vi "LtaSet.vi"(8 "Error In":errorcluster[](array[cluster]), 10 "Data":variant) -> (0 "Error Out":errorcluster[](array[cluster]), 2 "BusNum":i32)   [LabVIEW 2014, in "Bus_class.lvlib" / "Bus.lvclass"]
uses:
  Bus.lvclass
  TestAutomation/Comms/CommsData.ctl
  <vilib>/Utility/error.llb/Error Cluster From Error Code.vi
  <vilib>/ErrorRing/Error Ring.xnode
  TestAutomation/Comms/Comms.lvlib
  <userlib>/NIST/NISTErrorLib/NISTErrorLib.lvlib
  TestAutomation/LTA/LTA.lvlib
  Framework.lvlib
panel:
  out "XMLData":string
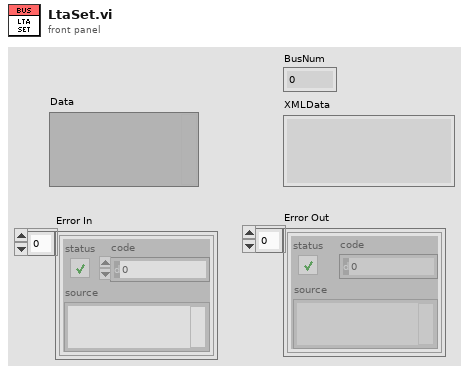
[diagram p1: front panel]
types:
  T1 = typedef "Comms.lvlib/CommsData.ctl" = cluster{"Command":string, "XMLData":string}
  T2 = typedef "Framework.lvlib/clFrameworkData.ctl" = cluster{"EvtINIFilePaths":path[], "BusClassInstances":refnum<class "Bus.lvclass">[], "PmuImpairINIFilePaths":path[], "FlagImpairINIFilePaths":path[], "NetImpairINIFilePaths":path[], "OutputToFileINIFilePaths":path[], "AppINIFilePaths":path[], "AppModuleID":i32, "OutputToFileID":i32}
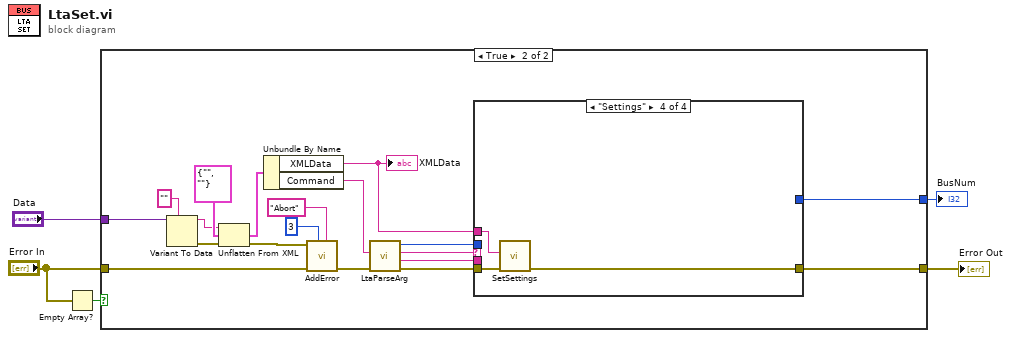
[diagram p0: block diagram]
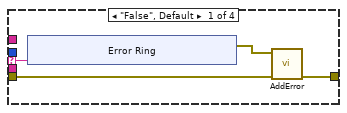
[diagram p3: hidden frame]
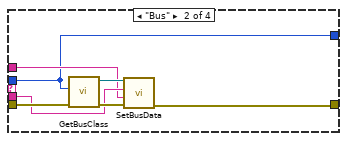
[diagram p4: hidden frame]
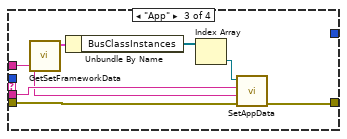
[diagram p5: hidden frame]
diagram:
  n1 = Empty Array?(array="Error In") -> (empty?=w5:bool)
  n2 = case shown="True" w5 {
    tunnel: "Error In" -> [w6 w17]
    tunnel: "Data" -> [_ w16]
    tunnel: [w6 w9] -> w2
    tunnel: [_ w7] -> w1
    frame False {
    }
    frame True {
      n3 = Variant To Data(type="", Variant=w16) -> (data=w20:string, error out=w19:errorcluster)  [unwired: 1 in]
      n4 = Unflatten From XML(xml string=w20, type=T1 {"Command"="", "XMLData"=""} ("CommsData"), error in (no error)=w19) -> (value=w25:T1, error out=w22:errorcluster)
      n5 = Unbundle By Name(w25) -> ("XMLData"=w8:string, "Command"=w12:string)
      "XMLData" <- w8
      n6 = call <userlib>:"AddError.vi"("Severity"="Abort", "Priority"=u8 3, "ErrorArray"=w17, "error in (no error)"=w22) -> ("ErrorArray"=w15:errorcluster[])  [unwired: 6 in, 1 out]
      n7 = call "LtaParseArg.vi"("Error In"=w15, "Arg In"=w12) -> ("Error Out"=w14:errorcluster[], "ArgRemaining"=w10:string, "Arg 1"=w11:string, "Arg1Num"=w13:i32)  [unwired: 6 in]
      n8 = case shown="\"Settings\"" w11 {
        selector: w11 -> [w29 _ _ _]
        tunnel: w14 -> [w27 w43 w47 w53]
        tunnel: w13 -> [_ w37 _ _]
        tunnel: w10 -> [_ w40 w50 _]
        tunnel: [w26 w38 w48 w52] -> w9
        tunnel: w8 -> [_ w39 w49 w51]
        tunnel: [_ w37 _ _] -> w7
        frame "False", Default {
          n9 = xnode "Error Ring"("parameter 0"=w29) -> ("error out"=w28:errorcluster)
          n10 = call <userlib>:"AddError.vi"("ErrorArray"=w27, "error in (no error)"=w28) -> ("ErrorArray"=w26:errorcluster[])  [unwired: 8 in, 1 out]
        }
        frame "Bus" {
          n11 = call "GetBusClass.vi"("ErrorArray In"=w43, "BusNumber"=w37) -> ("ErrorArray Out"=w42:errorcluster[], "Framework.lvlib:Bus.lvclass"=w41:refnum<class "Bus.lvclass">)  [unwired: 8 in]
          n12 = call "SetBusData.vi"("Error In"=w42, "XmlData"=w39, "arg"=w40, "Bus in"=w41) -> ("Error Out"=w38:errorcluster[])  [unwired: 6 in, 1 out]
        }
        frame "App" {
          n13 = call "GetSetFrameworkData.vi"() -> ("clFrameworkData Out"=w46:T2)  [unwired: 11 in]
          n14 = Unbundle By Name(w46) -> ("BusClassInstances"=w44:refnum<class "Bus.lvclass">[])
          n15 = Index Array(array=w44) -> (element=w45:refnum<class "Bus.lvclass">)  [unwired: 1 in]
          n16 = call "SetAppData.vi"("Error In"=w47, "XmlData"=w49, "arg"=w50, "Bus in"=w45) -> ("Error Out"=w48:errorcluster[])  [unwired: 6 in, 1 out]
        }
        frame "Settings" {
          n17 = call "SetSettings.vi"("Error In"=w53, "XmlData"=w51) -> ("Error Out"=w52:errorcluster[])  [unwired: 9 in]
        }
      }
    }
  }
  "Error Out" <- w2
  "BusNum" <- w1
